vi "TDMS path from Experiment Folder.vi"(8 "error in (no error)":errorcluster, 11 "experiment folder":path) -> (0 "error out":errorcluster, 2 "name":string, 3 "tdms file path":path)   [LabVIEW 2016]
uses:
  <userlib>/_OpenG.lib/file/file.llb/Strip Path - Traditional__ogtk.vi
  <userlib>/_OpenG.lib/file/file.llb/Build Path - Traditional__ogtk.vi
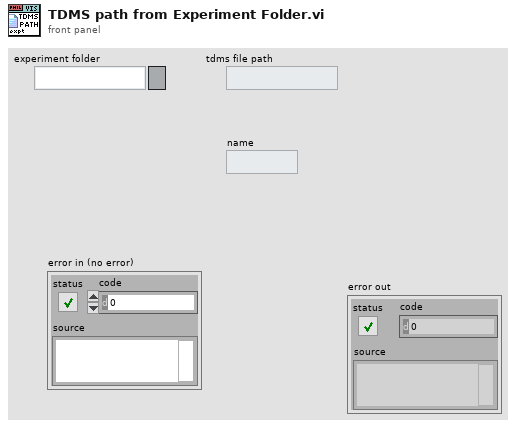
[diagram p1: front panel]
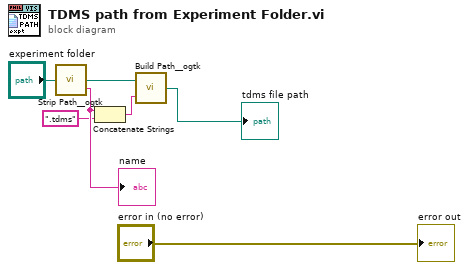
[diagram p0: block diagram]
diagram:
  n1 = call-poly <userlib>:"Strip Path__ogtk.vi"("path"="experiment folder") -> ("stripped path"=w3:path, "name"=w7:string)
  "name" <- w7
  n2 = Concatenate Strings(w7, ".tdms" ("string")) -> (w4:string)
  n3 = call-poly <userlib>:"Build Path__ogtk.vi"("name or relative path"=w4, "base path"=w3) -> ("appended path"=→"tdms file path":path)
  "error out" <- "error in (no error)"
